vi "Disconnect.vi"(8 "error in (no error)":errorcluster, 11 "FTPProtocol in":refnum<class "FTPProtocol.lvclass">) -> (0 "error out":errorcluster, 3 "FTPProtocol out":refnum<class "FTPProtocol.lvclass">)   [LabVIEW 2020, in "FileSync -- FTP.lvlib" / "FTPProtocol.lvclass"]
uses:
  FTPProtocol.lvclass
  FTPProtocol.lvclass/FTPProtocol.ctl
  _support/FTP Toolkit/FTP Class/FTP.lvclass
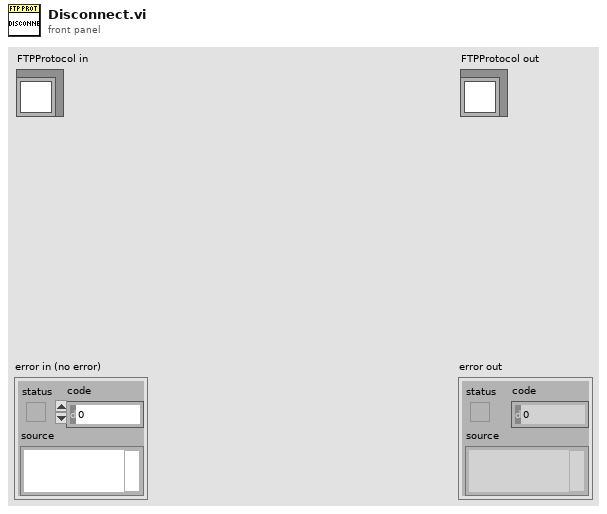
[diagram p1: front panel]
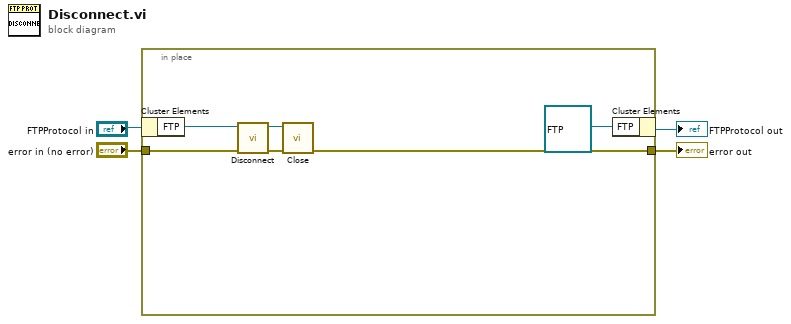
[diagram p0: block diagram]
diagram:
  n1 = in-place "In Place Element Structure" {
    in-place-border: "error in (no error)" -> [w6]
    in-place-border: [w5] -> w1
    n2 = in-place-cluster #1("FTPProtocol in") -> ("FTP"=w7:refnum<class "FTP.lvclass">)
    n3 = call "Disconnect.vi"("error in (no error)"=w6, "FTP in"=w7) -> ("error out"=w8:errorcluster, "FTP out"=w9:refnum<class "FTP.lvclass">)  [unwired: 8 in]
    n4 = call "Close.vi"("error in (no error)"=w8, "FTP in"=w9) -> ("error out"=w5:errorcluster)  [unwired: 9 in]
    n5 = in-place-cluster #1("FTP"=refnum<class "FTP.lvclass"> refnum ("FTP out")) -> (→"FTPProtocol out":refnum<class "FTPProtocol.lvclass">)
  }
  "error out" <- w1
